vi "Simple Add Subtract.vi"() -> ()   [LabVIEW 2020, in "OPI.lvclass"]
uses:
  OPI.lvclass
  Typedefs/Cmd Line Mode.ctl
  Set Arguments/Set Argument - Float.vi
  Get Return/Get Return - Float.vi
panel:
  in  "Stop":bool
  out "Add Return":dbl=10.0
  out "Subtract Return":dbl=-2.0
  in  "In2":dbl=6.0
  in  "In1":dbl=4.0
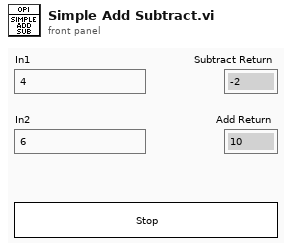
[diagram p1: front panel]
types:
  T1 = typedef "OPI.lvclass/Cmd Line Mode.ctl" = enum16{"Debug", "Hidden"}
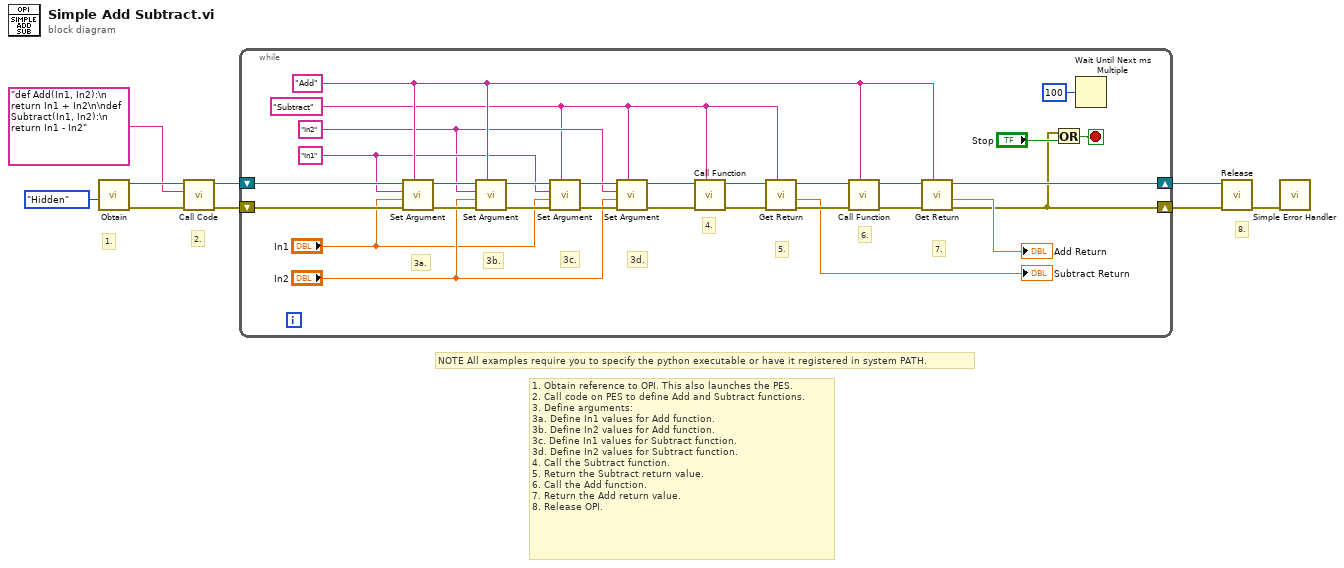
[diagram p0: block diagram]
diagram:
  # "NOTE All examples require you to specify the python executable or have it registered in system PATH."
  # "1. Obtain reference to OPI. This also launches the PES.\n2. Call code on PES to define Add and Subtract functions.\n3. Define arguments:\n3a. Define In1 values for Add function.\n3b. Define In2 values for Add function.\n3c. Define In1 values for Subtract function.\n3d. Define In2 values for Subtract function.\n4. Call the Subtract function.\n5. Return the Subtract return value.\n6. Call the Add function.\n7. Return the Add return value.\n8. Release OPI."
  # "8."
  # "2."
  # "1."
  n1 = call "Obtain.vi"("Cmd Line Mode (Hidden)"=Cmd_Line_Mode."Hidden") -> ("Error Out"=w8:errorcluster, "OPI Ref"=w9:refnum<data-value>)  [unwired: 9 in]
  n2 = call "Call Code.vi"("Error In"=w8, "Pythonic Code"="def Add(In1, In2):\n    return In1 + In2\n\ndef Subtract(In1, In2):\n    return In1 - In2", "OPI Ref"=w9) -> ("Error Out"=w5:errorcluster, "OPI Ref"=w6:refnum<data-value>)  [unwired: 7 in]
  n3 = while {
    shift-right: [w15] -> w4
    shift-left: w6 -> [w35]
    shift-right: [w12] -> w2
    shift-left: w5 -> [w34]
    stop <- w38 stop-if-true
    w25 = "In2" ("Argument")
    w26 = "In1" ("Argument")
    w18 = "Subtract" ("Function")
    w32 = "Add" ("Function")
    # "7."
    # "6."
    # "5."
    # "4."
    # "3d."
    # "3c."
    # "3b."
    # "3a."
    n4 = call-poly "Set Argument.vi"("Function Name"=w32, "Error In"=w34, "Float"="In1", "Argument"=w26, "OPI Ref"=w35) -> ("Error Out"=w31:errorcluster, "OPI Ref"=w33:refnum<data-value>)  [unwired: 5 in]
    n5 = call-poly "Set Argument.vi"("Function Name"=w32, "Error In"=w31, "Float"="In2", "Argument"=w25, "OPI Ref"=w33) -> ("Error Out"=w27:errorcluster, "OPI Ref"=w30:refnum<data-value>)  [unwired: 5 in]
    n6 = call-poly "Set Argument.vi"("Function Name"=w18, "Error In"=w27, "Float"="In1", "Argument"=w26, "OPI Ref"=w30) -> ("Error Out"=w28:errorcluster, "OPI Ref"=w29:refnum<data-value>)  [unwired: 5 in]
    n7 = call-poly "Set Argument.vi"("Function Name"=w18, "Error In"=w28, "Float"="In2", "Argument"=w25, "OPI Ref"=w29) -> ("Error Out"=w23:errorcluster, "OPI Ref"=w24:refnum<data-value>)  [unwired: 5 in]
    n8 = call "Call Function.vi"("Function Name"=w18, "Error In"=w23, "OPI Ref"=w24) -> ("Error Out"=w21:errorcluster, "OPI Ref"=w22:refnum<data-value>)  [unwired: 7 in]
    n9 = call-poly "Get Return.vi"("Function Name"=w18, "Error In"=w21, "OPI Ref"=w22) -> ("Error Out"=w19:errorcluster, "Float"=→"Subtract Return":dbl, "OPI Ref"=w20:refnum<data-value>)  [unwired: 6 in]
    n10 = call "Call Function.vi"("Function Name"=w32, "Error In"=w19, "OPI Ref"=w20) -> ("Error Out"=w36:errorcluster, "OPI Ref"=w37:refnum<data-value>)  [unwired: 7 in]
    n11 = call-poly "Get Return.vi"("Function Name"=w32, "Error In"=w36, "OPI Ref"=w37) -> ("Error Out"=w12:errorcluster, "Float"=→"Add Return":dbl, "OPI Ref"=w15:refnum<data-value>)  [unwired: 6 in]
    n12 = Or(x=w12, y="Stop") -> (x .or. y?=w38:bool)
    n13 = Wait Until Next ms Multiple(millisecond multiple=u32 100) -> ()  [unwired: 1 out]
  }
  n14 = call "Release.vi"("Error In"=w2, "OPI Ref"=w4) -> ("Error Out"=w1:errorcluster)  [unwired: 9 in]
  n15 = call <vilib>:"Simple Error Handler.vi"("error in (no error)"=w1) -> ()  [unwired: 4 in, 5 out]
